vi "GDSString_AttributeTextToAttributeType.vi"(9 "MethodText":string, 10 "DefaultAccessScope(Private)":T1=enum."private", 11 "AttributeText":string) -> (0 "ClassesOrTypesDependency":string[](array[string]), 1 "Structs":T2[](array[typedef]), 2 "Enums":T6[](array[typedef]), 3 "Attributes":T4[](array[typedef]))   [LabVIEW 2012]
uses:
  CommonVIs/CommonVIs_AttributeType.ctl
  <resource>/Framework/Providers/Open_GDS/ClassProviders/Common/CommonVIs/CommonVIs_AttributeDataType.ctl
  GDSString_AccessScopeModifierType.ctl
  CommonVIs/CommonVIs_EnumType.ctl
  GDSString_ModifierType.ctl
  CommonVIs/CommonVIs_StructType.ctl
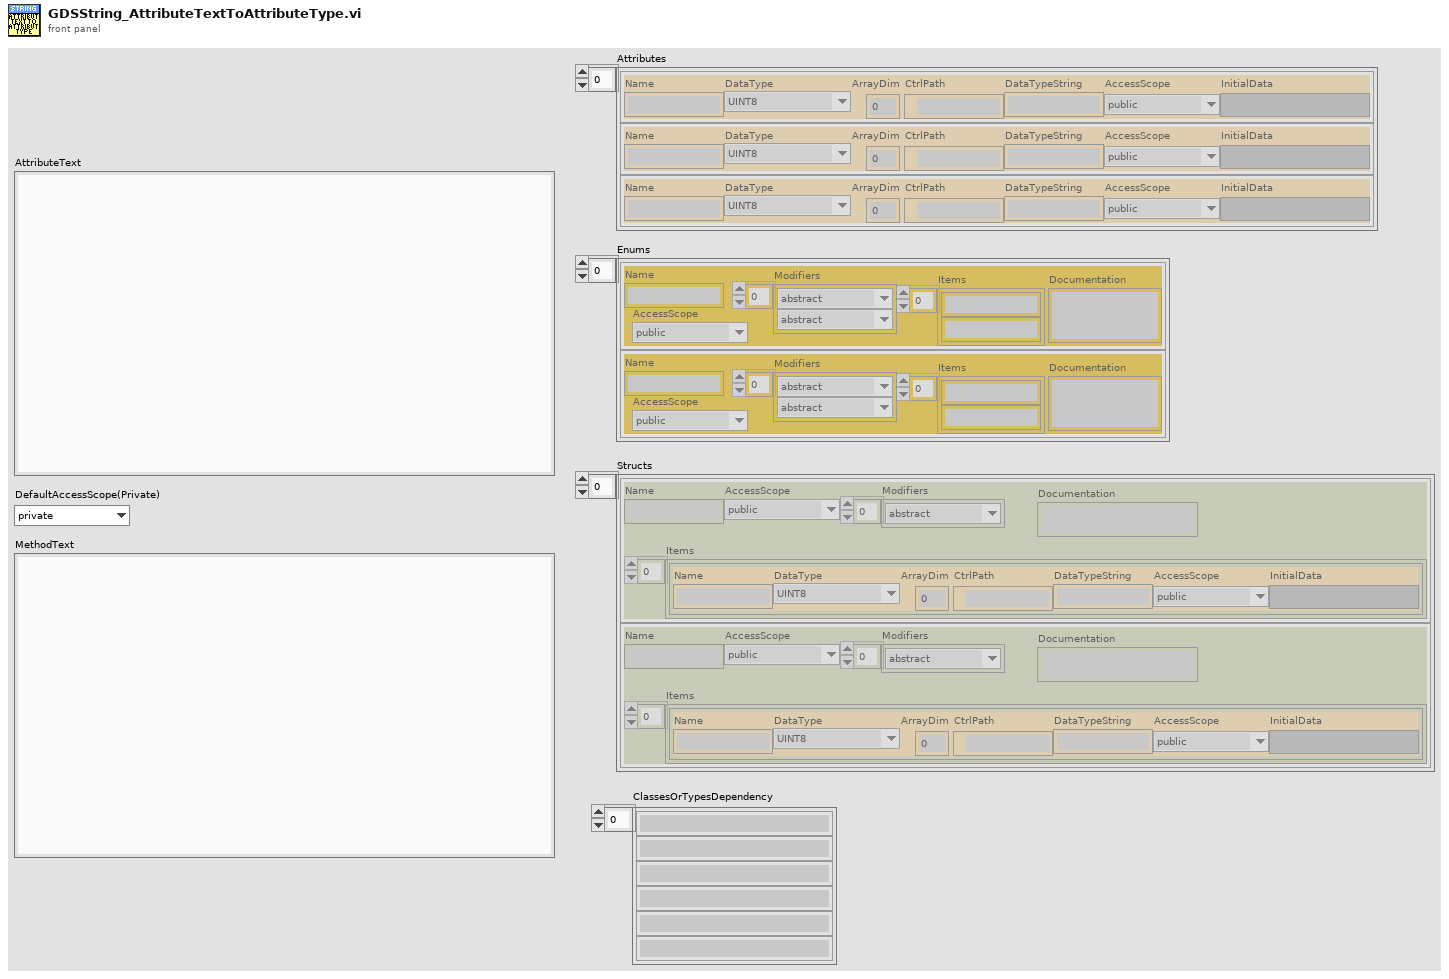
[diagram p1: front panel]
types:
  T1 = typedef "GDSString_AccessScopeModifierType.ctl" = enum16{"public", "private", "protected", "internal"}
  T2 = typedef "CommonVIs_StructType.ctl" = cluster{"Name":string, "AccessScope":T1, "Modifiers":T3[], "Items":T4[], "Documentation":string}
  T3 = typedef "GDSString_ModifierType.ctl" = enum16{"abstract", "static", "final", "synchronized", "strictfp", "async", "const", "event", "extern", "new", "override", "partial", "readonly", "sealed", "unsafe", "virtual", "volatile"}
  T4 = typedef "CommonVIs_AttributeType.ctl" = cluster{"Name":string, "DataType":T5, "ArrayDim":i32, "CtrlPath":path, "DataTypeString":string, "AccessScope":T1, "InitialData":variant}
  T5 = typedef "CommonVIs_AttributeDataType.ctl" = enum16{"UINT8", "INT8", "UINT16", "INT16", "UINT32", "INT32", "UINT64", "INT64", "SGL", "DBL", "EXT", "CSG", "CDB", "CXT", "TimeStamp", "STRING", "PATH", "BOOL", "ENUM", "RefNum", "VIRefNum", "ClassRefNum", "Cluster", "Variant", "TypeRef", "Waveform", "LabVIEW Object", "Other", "void"}
  T6 = typedef "CommonVIs_EnumType.ctl" = cluster{"Name":string, "AccessScope":T1, "Modifiers":T3[], "Items":string[], "Documentation":string}
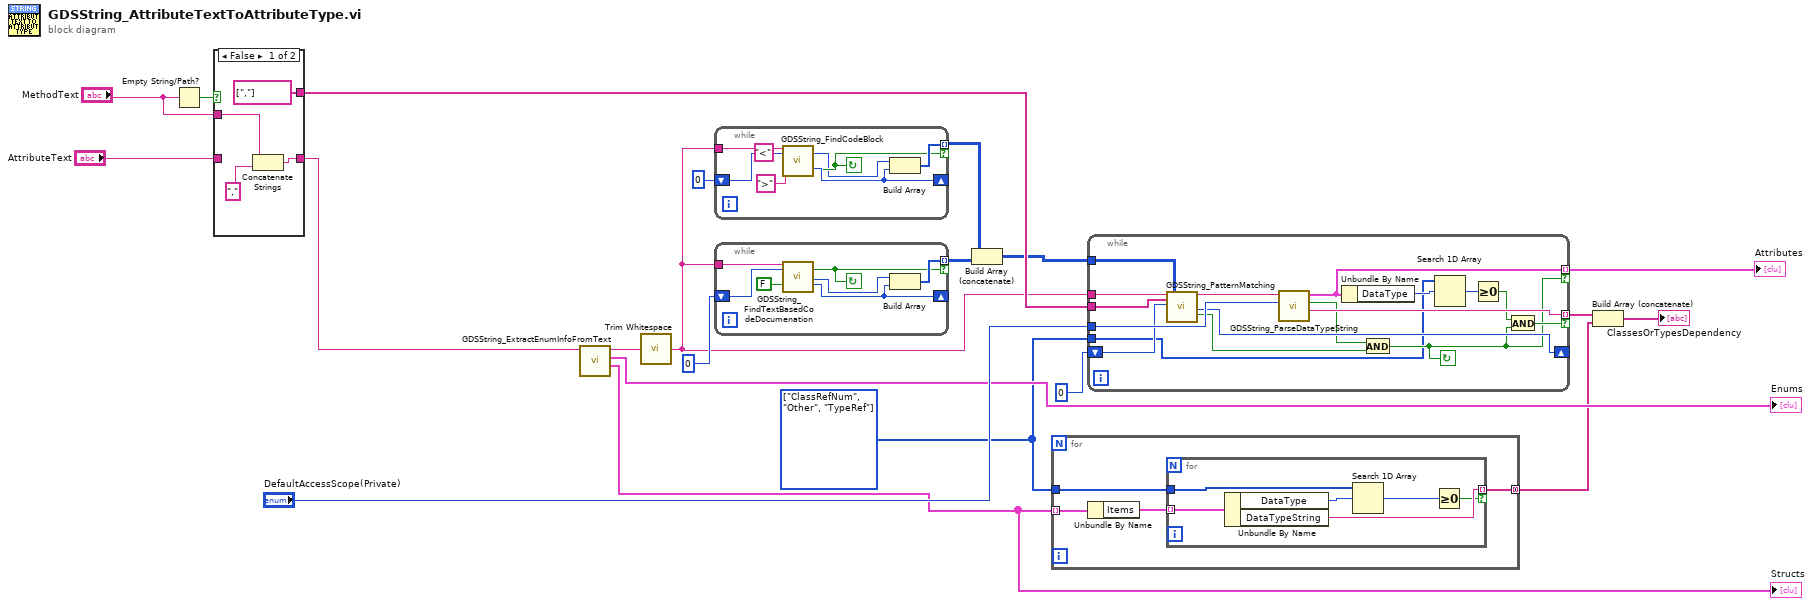
[diagram p0: block diagram]
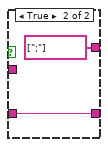
[diagram p2: hidden frame]
diagram:
  w11 = T5[] [enum."ClassRefNum", enum."Other", enum."TypeRef"] items=["UINT8", "INT8", "UINT16", "INT16", "UINT32", "INT32", "UINT64", "INT64", "SGL", "DBL", "EXT", "CSG", "CDB", "CXT", "TimeStamp", "STRING", "PATH", "BOOL", "ENUM", "RefNum", "VIRefNum", "ClassRefNum", "Cluster", "Variant", "TypeRef", "Waveform", "LabVIEW Object", "Other", "void"] ("1D array")
  n1 = Empty String/Path?(string/path="MethodText") -> (empty?=w8:bool)
  n2 = case shown="False" w8 {
    tunnel: [string[] [","] ("PatternMatchingStrings") string[] [";"] ("PatternMatchingStrings")] -> w16
    tunnel: "MethodText" -> [w24 _]
    tunnel: [w23 w26] -> w5
    tunnel: "AttributeText" -> [_ w26]
    frame False {
      n3 = Concatenate Strings(w24, "," ("regular expression")) -> (w23:string)
    }
    frame True {
    }
  }
  n4 = call "GDSString_ExtractEnumInfoFromText.vi"("AttributeStringIn"=w5) -> ("Structs"=w12:T2[], "Enums"=→"Enums":T6[], "StructsAndEnumsRemoved"=w15:string)  [unwired: 7 in, 1 out]
  "Structs" <- w12
  n5 = call <vilib>:"Trim Whitespace.vi"("string"=w15) -> ("trimmed string"=w3:string)  [unwired: 1 in]
  n6 = while {
    tunnel: w3 -> [w35]
    shift-right: [w34] -> _
    shift-left: 0 ("offset past match") -> [w33]
    tunnel: [w32] -> w1 mode=indexing if=w31
    stop <- w31 continue-if-true
    n7 = call "GDSString_FindCodeBlock.vi"("Text"=w35, "StringStartOffset(Default=-1 => 0 for Forward, StrLenght for Backwards)"=w33, "CodeBlockStartCharacter( { )"="<", "CodeBlockEndCharacter( } )"=">") -> ("found"=w31:bool, "BlockStart(Outside)"=w28:i32, "BlockEnd(Outside)"=w34:i32)  [unwired: 7 in, 6 out]
    n8 = Build Array(w28, w34) -> (w32:i32[])
  }
  n9 = while {
    tunnel: w3 -> [w42]
    shift-right: [w40] -> _
    shift-left: 0 ("offset past match") -> [w39]
    tunnel: [w38] -> w13 mode=indexing if=w37
    stop <- w37 continue-if-true
    n10 = call "GDSString_FindTextBasedCodeDocumenation.vi"("Text"=w42, "StringStartOffset(Default=-1 => 0 for Forward, StrLenght for Backwards)"=w39, "CommentHasToBeTheFirstItem(True)"=FALSE) -> ("Found"=w37:bool, "IndexBeforeDocument(Or after when searching Backwards)"=w41:i32, "IndexAfterDocument(Or before when searching Backwards)"=w40:i32)  [unwired: 12 in, 2 out]
    n11 = Build Array(w41, w40) -> (w38:i32[])
  }
  n12 = Build Array (concatenate)(w1, w13) -> (w2:i32[][])
  n13 = for {
    tunnel: w12 -> [w46] mode=indexing
    tunnel: w11 -> [w44]
    tunnel: [w43] -> w10 mode=concatenating
    n14 = Unbundle By Name(w46) -> ("Items"=w45:T4[])
    n15 = for {
      tunnel: w45 -> [w52] mode=indexing
      tunnel: w44 -> [w49]
      tunnel: [w48] -> w43 mode=indexing if=w47
      n16 = Unbundle By Name(w52) -> ("DataType"=w50:T5, "DataTypeString"=w48:string)
      n17 = Search 1D Array(1D array=w49, element=w50) -> (index of element=w51:i32)  [unwired: 1 in]
      n18 = Greater Or Equal To 0?(x=w51) -> (x >= 0?=w47:bool)
    }
  }
  n19 = while {
    tunnel: [w63] -> w21 mode=indexing if=w55
    tunnel: "DefaultAccessScope(Private)" -> [w68]
    tunnel: [w67] -> w20 mode=indexing if=w64
    tunnel: w16 -> [w61]
    tunnel: w3 -> [w60]
    shift-right: [w58] -> _
    shift-left: 0 ("offset past match") -> [w59]
    tunnel: w2 -> [w53]
    tunnel: w11 -> [w54]
    stop <- w55 continue-if-true
    n20 = call "GDSString_PatternMatching.vi"("TextIn"=w60, "PatternMatchingStrings"=w61, "StringStartOffset(Default=-1 => 0 for Forward, StrLenght for Backwards)"=w59, "IgnoreMatchesWithinThesePositions"=w53) -> ("TextBefore"=w69:string, "IndexAfterMatch(Or before when searching Backwards)"=w58:i32, "Found"=w57:bool)  [unwired: 9 in, 4 out]
    n21 = call "GDSString_ParseDataTypeString.vi"("DefaultAccessScope(Private)"=w68, "InputText"=w69) -> ("DataTypeString"=w67:string, "Found"=w56:bool, "DataType"=w63:T4)  [unwired: 7 in]
    n22 = Unbundle By Name(w63) -> ("DataType"=w62:T5)
    n23 = And(x=w56, y=w57) -> (x .and. y?=w55:bool)
    n24 = Search 1D Array(1D array=w54, element=w62) -> (index of element=w66:i32)  [unwired: 1 in]
    n25 = Greater Or Equal To 0?(x=w66) -> (x >= 0?=w65:bool)
    n26 = And(x=w65, y=w55) -> (x .and. y?=w64:bool)
  }
  "Attributes" <- w21
  n27 = Build Array (concatenate)(w20, w10) -> (→"ClassesOrTypesDependency":string[])
